vi "GeneratePiezoRampWaveform.vi"(7 "Waveform Type":enum16{"Triangle", "Sawtooth"}(ring), 9 "Delta":dbl, 10 "Min":dbl, 11 "Max":dbl) -> (1 "Volume Size":i32, 2 "Volume Number":dbl[](array[numeric]), 3 "Ramp":dbl[](array[numeric]))   [LabVIEW 2015]
uses:
  NIDAQControls/NIDAQGlobals.vi
panel:
  out "Waveform Graph":dbl[](graph)
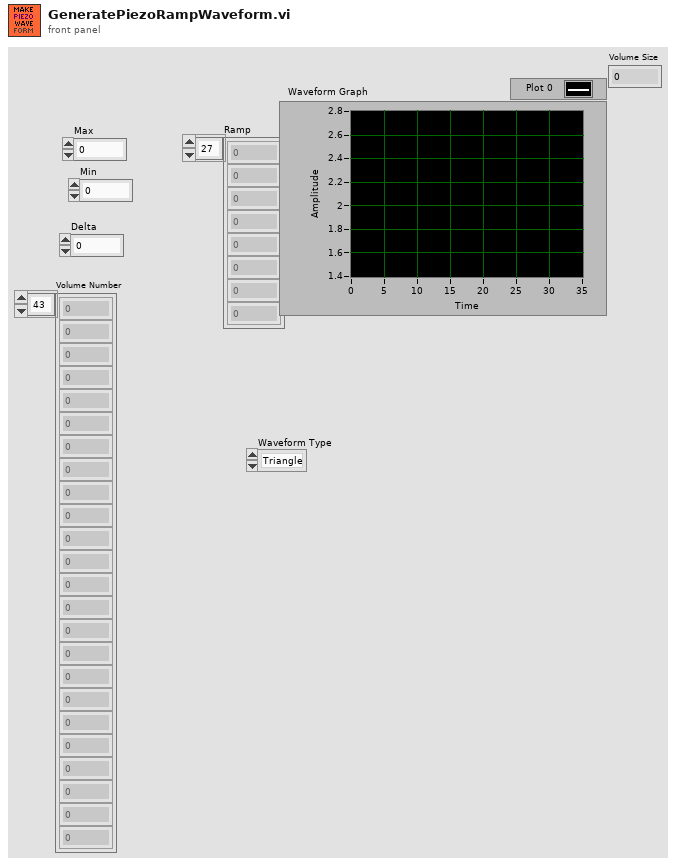
[diagram p1: front panel]
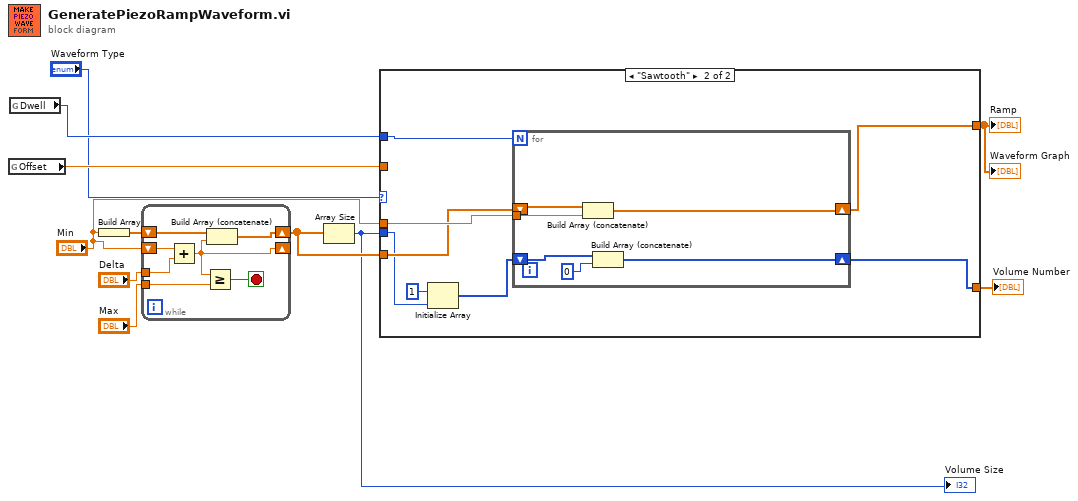
[diagram p0: block diagram]
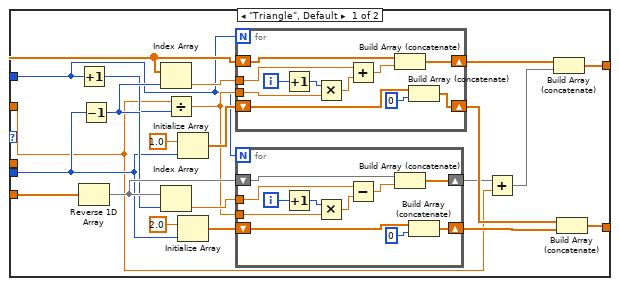
[diagram p2: hidden frame]
diagram:
  n1 = global read "NIDAQGlobals.vi" "Offset"() -> (w3:dbl)
  n2 = global read "NIDAQGlobals.vi" "Dwell"() -> (w4:u16)
  n3 = Build Array("Min") -> (w7:dbl[])
  n4 = while {
    tunnel: "Max" -> [w14]
    shift-right: [w15] -> w9
    shift-left: w7 -> [w16]
    tunnel: "Delta" -> [w17]
    shift-right: [w12] -> _
    shift-left: "Min" -> [w18]
    stop <- w13 stop-if-true
    n5 = Add(x=w18, y=w17) -> (x+y=w12:dbl)
    n6 = Greater Or Equal?(x=w12, y=w14) -> (x >= y?=w13:bool)
    n7 = Build Array (concatenate)(w16, w12) -> (w15:dbl[])
  }
  n8 = Array Size(array=w9) -> (size(s)=w6:i32)
  "Volume Size" <- w6
  n9 = case shown="\"Sawtooth\"" "Waveform Type" {
    tunnel: w9 -> [w39 w67]
    tunnel: [w33 w62] -> w8
    tunnel: w6 -> [w30 w66]
    tunnel: [w25 w63] -> w5
    tunnel: w4 -> [w20 w69]
    tunnel: w3 -> [w19 _]
    tunnel: "Min" -> [_ w68]
    frame "Triangle", Default {
      n10 = Increment(x=w20) -> (x+1=w21:u16)
      n11 = Reverse 1D Array(array=w39) -> (reversed array=w38:dbl[])
      n12 = Decrement(x=w30) -> (x-1=w35:i32)
      n13 = Index Array(array=w39, index=w35) -> (element=w36:dbl)
      n14 = Index Array(array=w38, index=w35) -> (element=w37:dbl)
      n15 = Divide(x=w19, y=w21) -> (x/y=w22:dbl)
      n16 = Initialize Array(1.0 ("element"), w30) -> (w28:dbl[])
      n17 = Initialize Array(2.0 ("element"), w30) -> (w29:dbl[])
      n18 = for {
        N: w20 -> [_]
        shift-right: [w60] -> w34
        shift-left: w39 -> [w61]
        tunnel: w36 -> [w54]
        shift-right: [w58] -> w26
        shift-left: w28 -> [w59]
        tunnel: w22 -> [w57]
        i -> [w56]
        n19 = Increment(x=w56) -> (x+1=w55:i32)
        n20 = Multiply(x=w55, y=w57) -> (x*y=w53:dbl)
        n21 = Add(x=w54, y=w53) -> (x+y=w52:dbl)
        n22 = Build Array (concatenate)(w61, w52) -> (w60:dbl[])
        n23 = Build Array (concatenate)(w59, 0) -> (w58:dbl[])
      }
      n24 = for {
        N: w20 -> [_]
        shift-right: [w49] -> w24
        shift-left: w38 -> [w50]
        tunnel: w37 -> [w42]
        shift-right: [w46] -> w27
        shift-left: w29 -> [w48]
        tunnel: w22 -> [w40]
        i -> [w43]
        n25 = Increment(x=w43) -> (x+1=w45:i32)
        n26 = Multiply(x=w45, y=w40) -> (x*y=w44:dbl)
        n27 = Subtract(x=w42, y=w44) -> (x-y=w41:dbl)
        n28 = Build Array (concatenate)(w50, w41) -> (w49:dbl[])
        n29 = Build Array (concatenate)(w48, 0) -> (w46:dbl[])
      }
      n30 = Add(x=w24, y=w19) -> (x+y=w23:dbl[])
      n31 = Build Array (concatenate)(w34, w23) -> (w33:dbl[])
      n32 = Build Array (concatenate)(w26, w27) -> (w25:dbl[])
    }
    frame "Sawtooth" {
      n33 = Initialize Array(u16 1 ("element"), w66) -> (w64:u16[])
      n34 = for {
        N: w69 -> [_]
        tunnel: w68 -> [w75]
        shift-right: [w71] -> w63
        shift-left: w64 -> [w73]
        shift-right: [w70] -> w62
        shift-left: w67 -> [w74]
        n35 = Build Array (concatenate)(w74, w75) -> (w70:dbl[])
        n36 = Build Array (concatenate)(w73, 0) -> (w71:i32[])
      }
    }
  }
  "Ramp" <- w8
  "Waveform Graph" <- w8
  "Volume Number" <- w5
